vi "rotate.vi"(10 "Array in":dbl[](array[numeric]), 11 "i":i32) -> (2 "Array out":dbl[](array[numeric]))   [LabVIEW 2015]
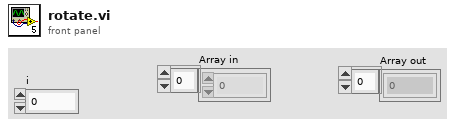
[diagram p1: front panel]
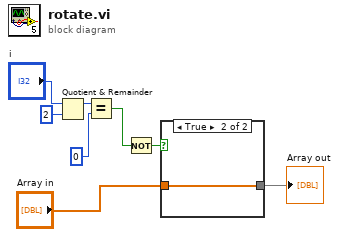
[diagram p0: block diagram]
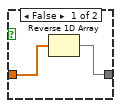
[diagram p2: hidden frame]
diagram:
  n1 = Quotient & Remainder(x="i", y=2) -> (x-y*floor(x/y)=w7:i32)  [unwired: 1 out]
  n2 = Equal?(x=w7, y=0) -> (x = y?=w1:bool)
  n3 = Not(x=w1) -> (.not. x?=w2:bool)
  n4 = case shown="True" w2 {
    tunnel: "Array in" -> [w10 w11]
    tunnel: [w9 w11] -> w4
    frame False {
      n5 = Reverse 1D Array(array=w10) -> (reversed array=w9:dbl[])
    }
    frame True {
    }
  }
  "Array out" <- w4
